vi "AIM664 Transmit Queue Write.vi"() -> ()   [LabVIEW 2020]
uses:
  src/AIM664LV.lvlib
panel:
  out "error out":errorcluster
  in  "Data":u8[](array[numeric])=[5, 2, 5, 6, 4, 5, 6, 7, 8, 9]
  out "BytesWritten":u32
  out "TxStatus":T1 {"TransmitMode" items=["FDX_TX_GENERIC", "FDX_TX_REPLAY", "FDX_TX_INDIVIDUAL"]; "TxStatus" items=["FDX_STAT_STOP", "FDX_STAT_RUN", "FDX_STAT_ERROR", "FDX_STAT_WAIT_F_TRIG"]}
  in  "UdpDescription":T2={"PortType"=1, "UdpSrc"=0, "IpSrc"=167846145, "VlId"=0, "IpDst"=3772776448, "UdpDst"=1, "SubVlId"=1, "UdpNumBufMessages"=5, "UdpMaxMessageSize"=800, "UdpSamplingRate"=0} {"IpDst" format="%x"; "IpSrc" format="%x"}
  in  "TransmitMode":u32(ring)=2 items=["FDX_TX_GENERIC", "FDX_TX_REPLAY", "FDX_TX_INDIVIDUAL"]
  in  "Input":T3={"VlId"=0, "SubVls"=4, "Bag"=8, "NetSelect"=3, "MaxFrameLength"=1000, "FrameBufferSize"=0, "MACSourceLSLW"=35520, "MACSourceMSLW"=512, "Skew"=0} {"MACSourceMSLW" format="%x"; "NetSelect" items=["FDX_TX_FRAME_DLY_A"=0, "FDX_TX_FRAME_DLY_B"=1, "FDX_TX_FRAME_BOTH "=3, "FDX_TX_FRAME_ONLY_A"=4, "FDX_TX_FRAME_ONLY_B "=5]; "MACSourceLSLW" format="%x"}
  out "ResourceInfo":T4 {"PortMode" items=[" FDX_SINGLE", "FDX_REDUNDANT"]}
  in  "TxControl":T5 {"ExtendedStopMode" items=["FDX_ESTOP_NOT_USED", "FDX_ESTOP_EXT_TRG", "FDX_ESTOP_EXT_TRG_RESTART", "FDX_ESTOP_TIME"]; "StartMode" items=["FDX_STOP", "FDX_START", "FDX_START_TRG", "FDX_START_TIME"]}
  in  "Input":T5={"StartMode"=1, "Count"=0, "Sign"=0, "Day"=0, "Hour"=0, "Min"=0, "Second"=0, "MilliSec"=0, "MicroSec"=0, "ExtendedStopMode"=0, "TransmitTime"=0} {"ExtendedStopMode" items=["FDX_ESTOP_NOT_USED", "FDX_ESTOP_EXT_TRG", "FDX_ESTOP_EXT_TRG_RESTART", "FDX_ESTOP_TIME"]; "StartMode" items=["FDX_STOP", "FDX_START", "FDX_START_TRG", "FDX_START_TIME"]}
  in  "Input Cluster":T6={"SrvName"="local", "ResourceID"=1, "ResourceType"=0} {"ResourceType" items=["Board", "Port"]}
  out "Output Cluster 2":T7={"ResourceID"=1, "ResourceType"=0, "ResourceInfo"="AMC-FDX-B2", "StructId"=0}
  in  "ServerRElement":u32=1
  out "PortInitOut":T8={"PortConfig"=0, "PortUsed"=1, "GlobalMemFree"=62889696, "SharedMemFree"=16566232} {"PortConfig" items=["FDX_SINGLE", "FDX_REDUNDANT"]}
  in  "ClientInfo":T9={"SrvName"="local", "ClHostName"="local", "ClUser"="Roland", "ClApplication"="Test", "ClApplicationVersion"="V01.00", "ResourceID"=2, "Privileges"=4294967295} {"Privileges" items=["PRIVILEGES_ADMIN"=4294967295]}
  out "NuOfResources":u32=3
  in  "SrvName":string="local"
  out "NuOfServers":u32=1
  # "ARINC 664 Transmit Queue Write"
  # "Overview: Configure the board to Transmit Data.\nRequirement: At least one AIM ARINC-664 board with installed AIM ARINC 664 BSP.\nRestrictions: None.\nInstruction:\n1. Run the VI.\n2. Verify the results in the indicators."
  # "QueryServerResourceCvi"
  # "FdxInitCvi"
  # "CountServerResourcesCvi"
  # "GetServerResourcesCvi"
  # "FdxLoginCvi"
  # "FdxTxPortInitCvi"
  # "FdxTxModeControlCvi"
  # "FdxTxCreateVLCvi"
  # "FdxTxUDPCreatePortCvi"
  # "FdxTxUDPWritePortCvi"
  # "FdxTxControlCvi"
  # "FdxTxStatusCvi"
  # "FdxTxControlCvi"
  # "Input"
  # "Input"
  # "Output"
  # "TxControl"
  # "Output"
  # "Output"
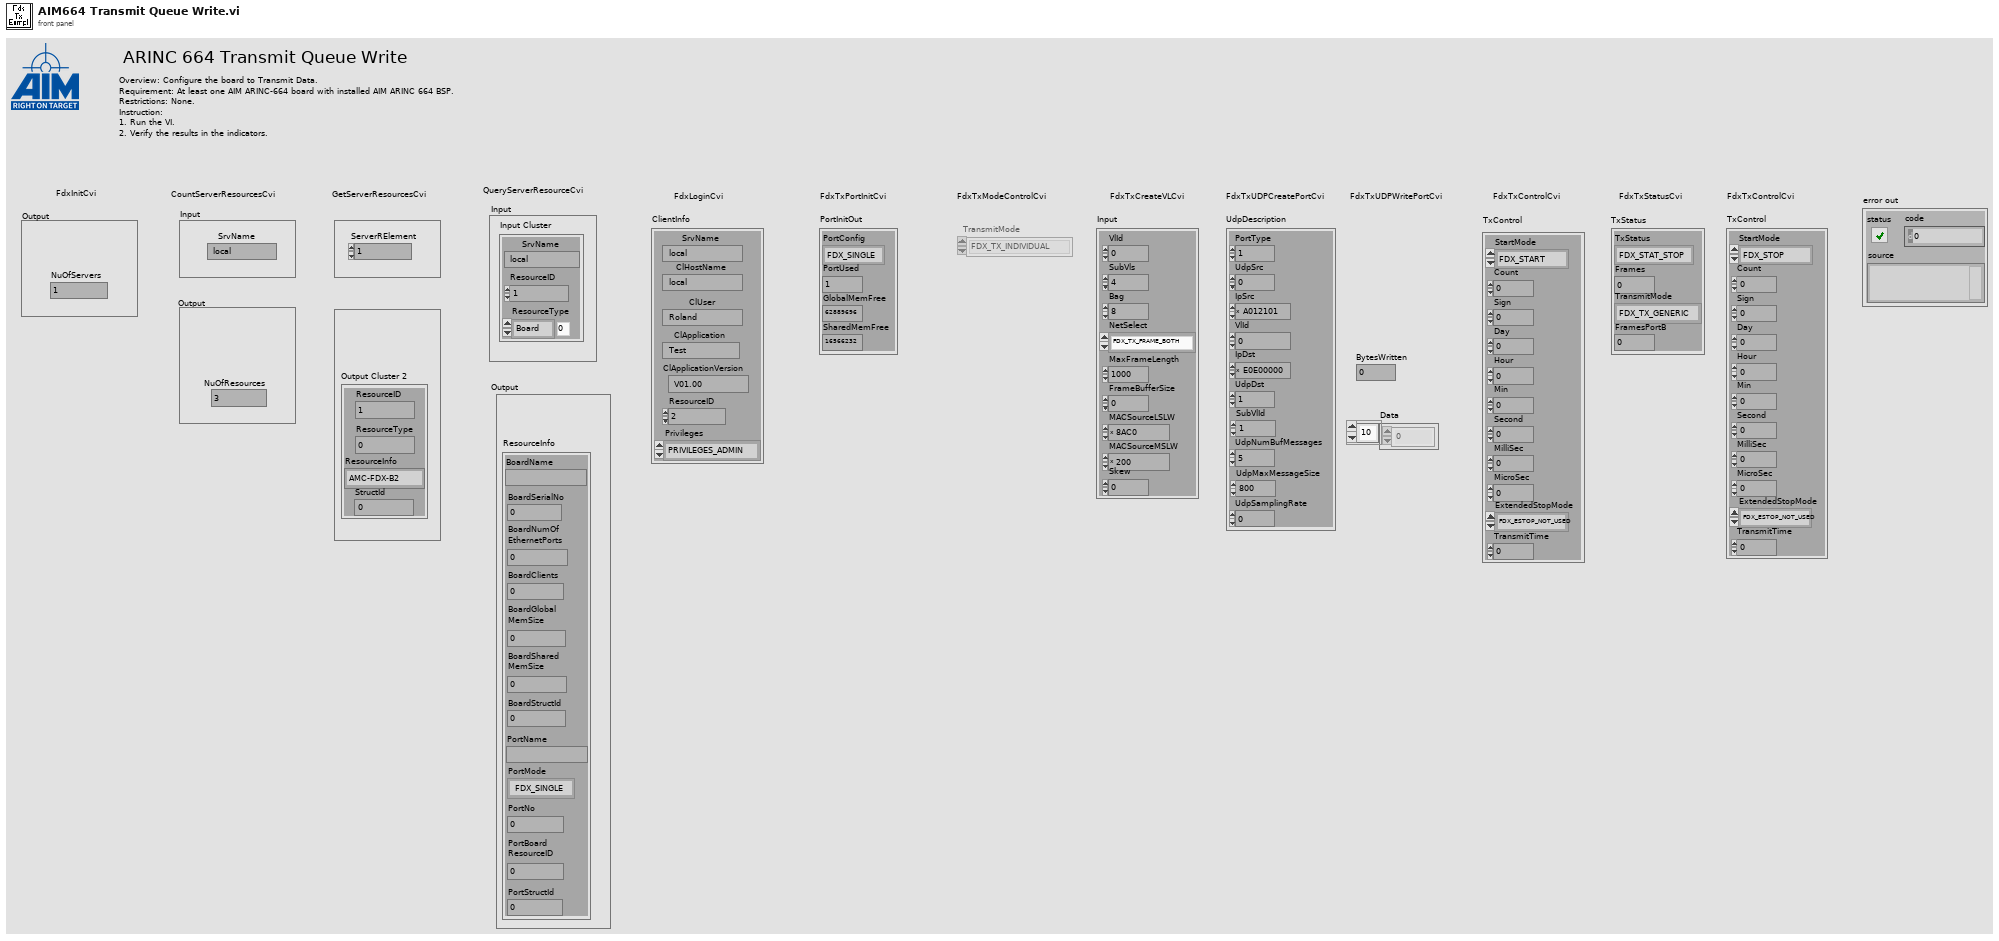
[diagram p1: front panel]
types:
  T1 = cluster{"TxStatus":u32, "Frames":u32, "TransmitMode":u32, "FramesPortB":u32}
  T2 = cluster{"PortType":u32, "UdpSrc":u32, "IpSrc":u32, "VlId":u32, "IpDst":u32, "UdpDst":u32, "SubVlId":u32, "UdpNumBufMessages":u32, "UdpMaxMessageSize":u32, "UdpSamplingRate":u32}
  T3 = cluster{"VlId":u32, "SubVls":u32, "Bag":u32, "NetSelect":u32, "MaxFrameLength":u32, "FrameBufferSize":u32, "MACSourceLSLW":u32, "MACSourceMSLW":u32, "Skew":u32}
  T4 = cluster{"BoardName":string, "BoardSerialNo":u32, "BoardNumOf\nEthernetPorts":u32, "BoardClients":u32, "BoardGlobal\nMemSize":u32, "BoardShared\nMemSize":u32, "BoardStructId":u32, "PortName":string, "PortMode":u32, "PortNo":u32, "PortBoard\nResourceID":u32, "PortStructId":u32}
  T5 = cluster{"StartMode":i32, "Count":u32, "Sign":i32, "Day":u32, "Hour":u32, "Min":u32, "Second":u32, "MilliSec":u32, "MicroSec":u32, "ExtendedStopMode":i32, "TransmitTime":u32}
  T6 = cluster{"SrvName":string, "ResourceID":u32, "ResourceType":u32}
  T7 = cluster{"ResourceID":u32, "ResourceType":u32, "ResourceInfo":string, "StructId":u32}
  T8 = cluster{"PortConfig":u32, "PortUsed":u32, "GlobalMemFree":u32, "SharedMemFree":u32}
  T9 = cluster{"SrvName":string, "ClHostName":string, "ClUser":string, "ClApplication":string, "ClApplicationVersion":string, "ResourceID":u32, "Privileges":u32}
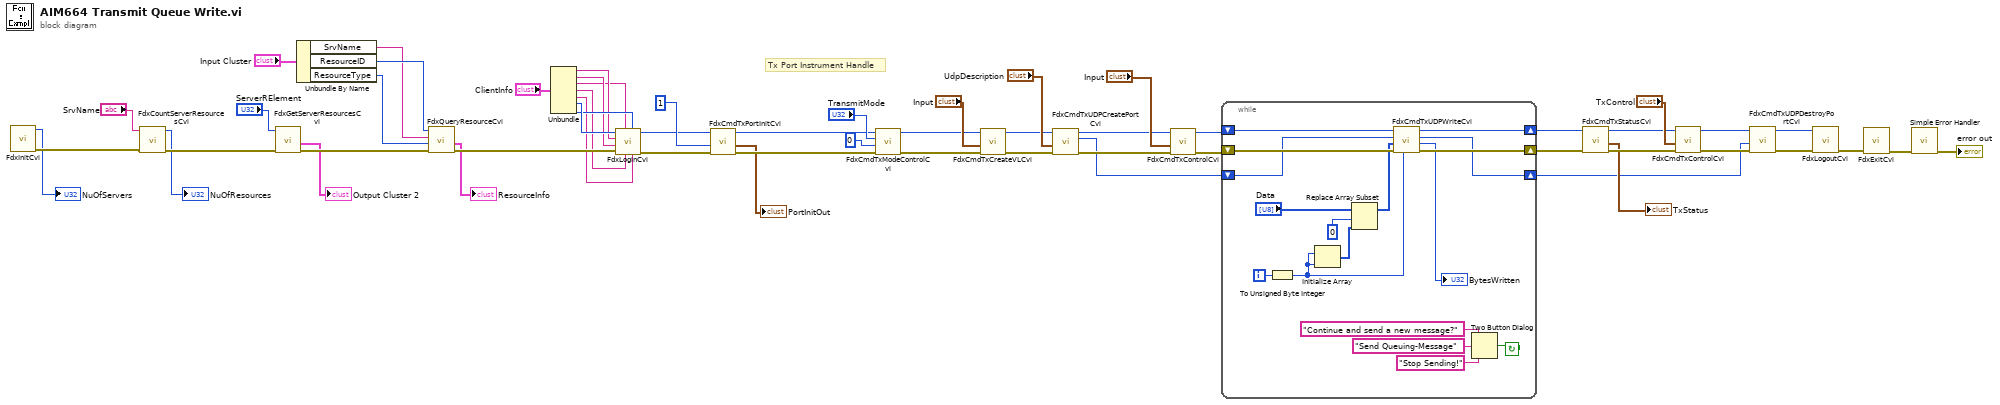
[diagram p0: block diagram]
diagram:
  # "Tx Port Instrument Handle"
  n1 = call "FdxInitCvi.vi"() -> ("error out"=w55:errorcluster, "Number of Servers"=→"NuOfServers":u32)  [unwired: 10 in]
  n2 = call "FdxCountServerResourcesCvi.vi"("error in"=w55, "SrvName (local)"="SrvName") -> ("error out"=w54:errorcluster, "Number of Resources"=→"NuOfResources":u32)  [unwired: 8 in]
  n3 = call "FdxGetServerResourcesCvi.vi"("error in"=w54, "ServerRElement"="ServerRElement") -> ("error out"=w49:errorcluster, "ServerResourceInfo"=→"Output Cluster 2":T7)  [unwired: 4 in, 4 out]
  n4 = Unbundle By Name("Input Cluster") -> ("SrvName"=w13:string, "ResourceID"=w14:u32, "ResourceType"=w12:u32)
  n5 = call "FdxQueryResourceCvi.vi"("error in"=w49, "ResourceType"=w12, "SrvName"=w13, "ResourceID"=w14) -> ("error out"=w42:errorcluster, "ResourceInfo"=→"ResourceInfo":T4)  [unwired: 5 in, 1 out]
  n6 = Unbundle("ClientInfo") -> ("SrvName"=w8:string, "ClHostName"=w7:string, "ClUser"=w6:string, "ClApplication"=w5:string, "ClApplicationVersion"=w4:string, "ResourceID"=w10:u32, "Privileges"=w9:u32)
  n7 = call "FdxLoginCvi.vi"("ClApplicationVersion"=w4, "Privileges"=w9, "ClApplication"=w5, "ClUser"=w6, "error in"=w42, "ClHostName"=w7, "SrvName"=w8, "ResourceID"=w10) -> ("error out"=w50:errorcluster, "InstrumentHandle"=w29:u32)  [unwired: 2 in]
  n8 = call "FdxCmdTxPortInitCvi.vi"("error in"=w50, "PortMap"=u32 1, "InstrumentHandle_port"=w29) -> ("error out"=w56:errorcluster, "PortInitOut"=→"PortInitOut":T8, "InstrumentHandle_port"=w28:u32)  [unwired: 6 in]
  n9 = call "FdxCmdTxModeControlCvi.vi"("error in"=w56, "RerosPortDelay"=u32 0, "TransmitMode"="TransmitMode", "InstrumentHandle_port"=w28) -> ("error out"=w52:errorcluster, "InstrumentHandle_port"=w27:u32)  [unwired: 6 in]
  n10 = call "FdxCmdTxCreateVLCvi.vi"("error in"=w52, "Input Cluster"="Input", "InstrumentHandle_port"=w27) -> ("error out"=w51:errorcluster, "InstrumentHandle_port"=w26:u32)  [unwired: 7 in]
  n11 = call "FdxCmdTxUDPCreatePortCvi.vi"("error in"=w51, "UdpDescription"="UdpDescription", "InstrumentHandle"=w26) -> ("error out"=w46:errorcluster, "UdpHandle"=w3:u32, "InstrumentHandle"=w25:u32)  [unwired: 6 in]
  n12 = call "FdxCmdTxControlCvi.vi"("error in"=w46, "TxControl"="Input", "InstrumentHandle_port"=w25) -> ("error out"=w47:errorcluster, "InstrumentHandle_port"=w24:u32)  [unwired: 7 in]
  n13 = while {
    shift-right: [w62] -> w23
    shift-left: w24 -> [w63]
    shift-right: [w60] -> w22
    shift-left: w3 -> [w61]
    shift-right: [w72] -> w43
    shift-left: w47 -> [w73]
    i -> [w65]
    stop <- w67 continue-if-true
    n14 = To Unsigned Byte Integer(number=w65) -> (unsigned 8bit integer=w57:u8)
    n15 = Initialize Array(w57, w57) -> (w64:u8[])
    n16 = Replace Array Subset(array="Data", new element=w64, index=0) -> (w58:u8[])
    n17 = call "FdxCmdTxUDPWriteCvi.vi"("ByteCount"=w57, "error in"=w73, "Data"=w58, "UdpHandle"=w61, "InstrumentHandle"=w63) -> ("error out"=w72:errorcluster, "BytesWritten"=→"BytesWritten":u32, "UdpHandle Out"=w60:u32, "InstrumentHandle"=w62:u32)  [unwired: 3 in]
    n18 = Two Button Dialog(message="Continue and send a new message?", 1:"Stop Sending!" ("F button name (\"Cancel\")"), 2:"Send Queuing-Message" ("T button name (\"OK\")")) -> (T button?=w67:bool)
  }
  n19 = call "FdxCmdTxStatusCvi.vi"("error in"=w43, "InstrumentHandle_port"=w23) -> ("error out"=w53:errorcluster, "TxStatus"=→"TxStatus":T1, "InstrumentHandle_port"=w21:u32)  [unwired: 7 in]
  n20 = call "FdxCmdTxControlCvi.vi"("error in"=w53, "TxControl"="TxControl", "InstrumentHandle_port"=w21) -> ("error out"=w45:errorcluster, "InstrumentHandle_port"=w20:u32)  [unwired: 7 in]
  n21 = call "FdxCmdTxUDPDestroyPortCvi.vi"("error in"=w45, "UdpHandle"=w22, "InstrumentHandle"=w20) -> ("error out"=w44:errorcluster, "InstrumentHandle"=w19:u32)  [unwired: 7 in]
  n22 = call "FdxLogoutCvi.vi"("error in"=w44, "InstrumentHandle"=w19) -> ("error out"=w48:errorcluster)  [unwired: 9 in]
  n23 = call "FdxExitCvi.vi"("error in"=w48) -> ("error out"=w2:errorcluster)  [unwired: 10 in]
  n24 = call <vilib>:"Simple Error Handler.vi"("error in (no error)"=w2) -> ("error out"=→"error out":errorcluster)  [unwired: 4 in, 4 out]
